vi "lsl create outlet.vi"(8 "error in (no error)":errorcluster, 9 "max_buffered":i32=360, 10 "chunk_size":i32, 11 "streaminfo":T2) -> (0 "error out":errorcluster, 3 "outlet":T1)   [LabVIEW 2019, in "Lab Streaming Layer.lvlib"]
doc: "extern LIBLSL_C_API lsl_outlet lsl_create_outlet(lsl_streaminfo info, int32_t chunk_size, int32_t max_buffered);"
uses:
  Lab Streaming Layer.lvlib
  Custom Controls/lsl_streaminfo.ctl
  Custom Controls/lsl_outlet.ctl
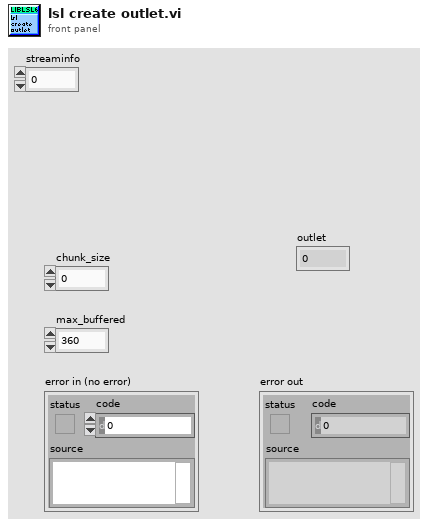
[diagram p1: front panel]
types:
  T1 = typedef "Lab Streaming Layer.lvlib/lsl_outlet.ctl" = u64
  T2 = typedef "Lab Streaming Layer.lvlib/lsl_streaminfo.ctl" = u64
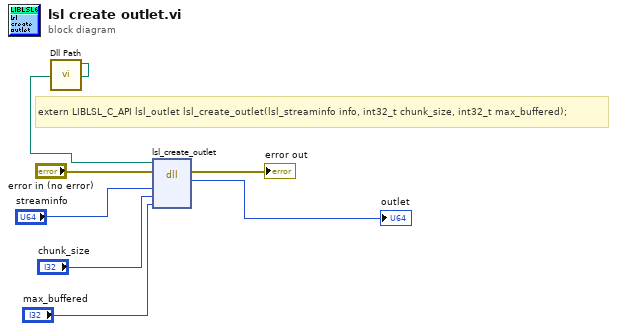
[diagram p0: block diagram]
diagram:
  # "extern LIBLSL_C_API lsl_outlet lsl_create_outlet(lsl_streaminfo info, int32_t chunk_size, int32_t max_buffered);"
  n1 = call "Dll Path.vi"() -> ("Dll path"=w1:path)  [unwired: 11 in]
  n2 = dll-call lib="E:/LabStreamingLayer/liblsl-LabVIEW-master/liblsl-LabVIEW-master/lsl.dll" fn="lsl_create_outlet"(path in=w1, error in="error in (no error)", "info"="streaminfo", "chunk_size"="chunk_size", "max_buffered"="max_buffered") -> (error out=→"error out":errorcluster, "return type"=→"outlet":u64)  [unwired: 4 in, 1 out]
